vi "Queue Comms Enqueue.vi"(8 "error in":errorcluster, 11 "element":T1={"Data"=variant, "Action"=enum."Exit"}) -> (0 "error out":errorcluster)   [LabVIEW 2025, in "Config Database.lvlib"]
doc: "This VI enqueues data. Should be swapped\nif different comms method used."
uses:
  Config Database.lvlib
  Private Controls/Module Data Cluster.ctl
  Private Controls/Module Action.ctl
  Private Controls/Queue FG Action.ctl
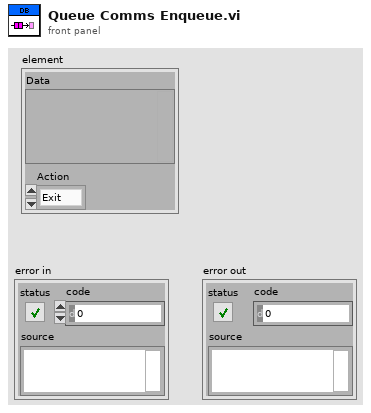
[diagram p1: front panel]
types:
  T1 = typedef "Config Database.lvlib/Module Data Cluster.ctl" = cluster{"Data":variant, "Action":T2}
  T2 = typedef "Config Database.lvlib/Module Action.ctl" = enum16{"Get balance", "Find Account", "Update balance", "Error", "Exit", "Init"}
  T3 = typedef "Config Database.lvlib/Queue FG Action.ctl" = enum16{"Release", "Get", "Set"}
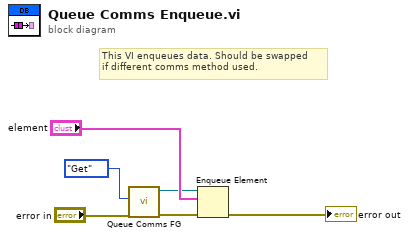
[diagram p0: block diagram]
diagram:
  # "This VI enqueues data. Should be swapped\nif different comms method used."
  n1 = call "Queue Comms FG.vi"("error in"="error in", "Action"=Queue_FG_Action."Get") -> ("error out"=w3:errorcluster, "Queue out"=w1:refnum<queue>)  [unwired: 8 in]
  n2 = Enqueue Element(queue=w1, element="element", error in (no error)=w3) -> (error out=→"error out":errorcluster)  [unwired: 1 in, 2 out]
